vi "F5xxx Initialize.vi"(8 "error in (no error)":errorcluster, 10 "Reset (False)":bool, 11 "session in":T1) -> (0 "error out":errorcluster, 2 "idn string":string, 3 "session out":T1)   [LabVIEW 2013]
doc: "Intialize and configurate Fluke 5xxx."
uses:
  F5xxx_session.ctl
  F5xxx_output_mode.ctl
  Fluke 5XXX Series Multicalibrators.lvlib
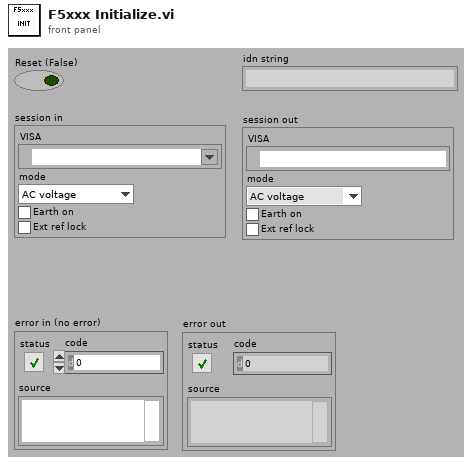
[diagram p1: front panel]
types:
  T1 = typedef "F5xxx_session.ctl" = cluster{"VISA":refnum<visa-resource-name>, "mode":T2, "Earth on":bool, "Ext ref lock":bool}
  T2 = typedef "F5xxx_output_mode.ctl" = enum16{"AC voltage", "AC current"}
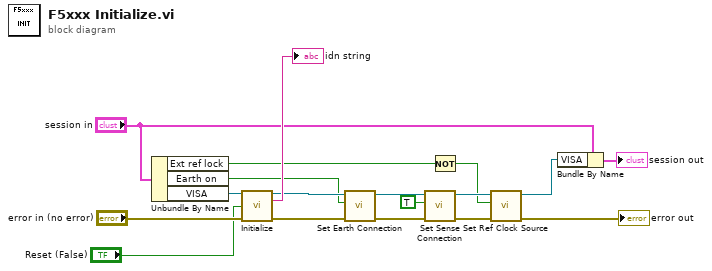
[diagram p0: block diagram]
diagram:
  n1 = Unbundle By Name("session in") -> ("Ext ref lock"=w6:bool, "Earth on"=w11:bool, "VISA"=w17:refnum<visa-resource-name>)
  n2 = call "Initialize.vi"("VISA resource name"=w17, "Reset (T: Reset)"="Reset (False)", "error in (no error)"="error in (no error)") -> ("VISA resource name out"=w13:refnum<visa-resource-name>, "idn string"=→"idn string":string, "error out"=w14:errorcluster)  [unwired: 10 in]
  n3 = call "Set Earth Connection.vi"("error in (no error)"=w14, "Earth Connection (F: Open)"=w11, "VISA resource name"=w13) -> ("error out"=w12:errorcluster, "VISA resource name out"=w10:refnum<visa-resource-name>)  [unwired: 7 in]
  n4 = call "Set Sense Connection.vi"("error in (no error)"=w12, "Sense Connection (T: Internal)"=TRUE, "VISA resource name"=w10) -> ("error out"=w8:errorcluster, "VISA resource name out"=w7:refnum<visa-resource-name>)  [unwired: 7 in]
  n5 = Not(x=w6) -> (.not. x?=w1:bool)
  n6 = call "Set Ref Clock Source.vi"("error in (no error)"=w8, "Reference Source (T: Internal)"=w1, "VISA resource name"=w7) -> ("error out"=→"error out":errorcluster, "VISA resource name out"=w3:refnum<visa-resource-name>)  [unwired: 7 in]
  n7 = Bundle By Name(cluster="session in", "VISA"=w3) -> (→"session out":T1)
